vi "Memory.Pointer.Clear Subset.vi"   [LabVIEW 2016, in "Memory Manager.lvlib" / "Memory.Pointer.lvclass"]
doc: "Sets the subset of bytes specified by <b>offset</b> and <b>length</b> within the provided <b>pointer</b> to zero."
uses:
  Memory.Pointer.lvclass
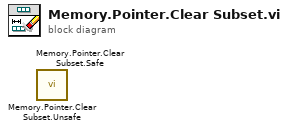
[diagram p0: block diagram]
diagram:
  n1 = call "Memory.Pointer.Clear Subset.Unsafe.vi"() -> ()  [unwired: 10 in, 2 out]
  n2 = call "Memory.Pointer.Clear Subset.Safe.vi"() -> ()  [unwired: 10 in, 2 out]
